vi "MouseWheelEvent.vi"(0 "reference in":refnum<class "LcPictureBox.lvclass">, 5 "error in (no error)":errorcluster) -> (14 "reference out":refnum<class "LcPictureBox.lvclass">, 15 "Event Callback Refnum":refnum<k27>, 16 "MouseWheelEvent":refnum<user-event>, 19 "error out":errorcluster)   [LabVIEW 2020, in "LcPictureBox.lvclass"]
uses:
  LcPictureBox.lvclass
  MouseWheelInfo.ctl
  System.Windows.Forms
  CallBackVIs/CallBack_MouseWheel.vi
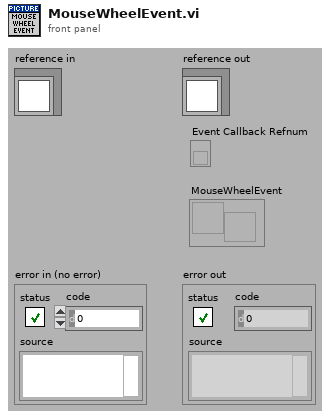
[diagram p1: front panel]
types:
  T1 = typedef "LcPictureBox.lvclass/MouseWheelInfo.ctl" = cluster{"X":i32, "Y":i32, "Button":i32, "Delta":i32, "X(raw)":i32, "Y(raw)":i32}
  T2 = typedef "LcPictureBox.lvclass/ObjectAttributes.ctl" = cluster{"PictureBox":refnum<k24>, "ImageSize":cluster{"Width":i32, "Height":i32}, "PenMemory":map{cluster{"Alpha(100%)":dbl, "Color(Black)":u32, "Pen(Width=1, Solid)":T3}, refnum<k24>}, "GraphicsRef":refnum<k24>, "BrushMemory":map{cluster{"Alpha(100%)":dbl, "Color(Black)":u32}, refnum<k24>}, "Images":refnum<k24>[], "ImageIndex":i32, "BgColor(None)":u32, "LoadedImages":map{string, cluster{"ImageOut":refnum<k24>, "ImageSize":cluster{"Width":i32, "Height":i32}}}, "ColorsMemory":map{cluster{"Alpha(100%)":dbl, "Color(Black)":u32}, refnum<k24>}, "CacheSize":i32, "PictureBoxActiveXReference":refnum<vi>, "Scale":sgl, "Offset":cluster{"x":sgl, "y":sgl}, "zoom_center":cluster{"X":i32, "Y":i32}, "ImagesCreated":refnum<k24>[]}
  T3 = typedef "LcPictureBox.lvclass/Pen.ctl" = cluster{"Width":u16, "Style":enum32{"Solid", "Dash", "Dot", "DashDot", "DashDotDot"}}
  T4 = cluster{"reference out":refnum<class "LcPictureBox.lvclass">, "MouseInfo":refnum<user-event>}
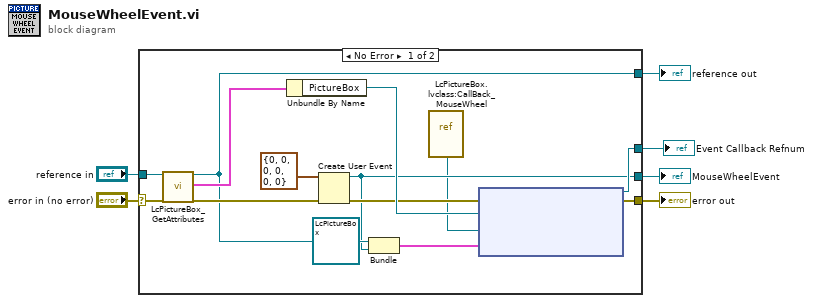
[diagram p0: block diagram]
diagram:
  n1 = case shown="No Error" "error in (no error)" {
    selector: "error in (no error)" -> [w19 w21]
    tunnel: [w13 w21] -> w5
    tunnel: [w10 w20] -> w3
    tunnel: "reference in" -> [w17 w20]
    tunnel: [w9 _] -> w1
    tunnel: [w12 _] -> w2
    frame No Error {
      (unwired) refnum<class "LcPictureBox.lvclass"> refnum ("reference out")
      n2 = call "LcPictureBox_GetAttributes.vi"("reference in"=w17, "error in (no error)"=w19) -> ("reference out"=w10:refnum<class "LcPictureBox.lvclass">, "Data"=w18:T2, "error out"=w14:errorcluster)  [unwired: 14 in, 1 out]
      n3 = Unbundle By Name(w18) -> ("PictureBox"=w16:refnum<k24>)
      n4 = Create User Event(user event datatype=T1 {"X"=0, "Y"=0, "Button"=0, "Delta"=0, "X(raw)"=0, "Y(raw)"=0} ("MouseInfo"), error in=w14) -> (user event=w9:refnum<user-event>, error out=w15:errorcluster)
      n5 = Bundle("reference out"=w10, "MouseInfo"=w9) -> (w7:T4)  [unwired: 1 in]
      n6 = vi-ref "LcPictureBox.lvclass:CallBack_MouseWheel.vi"() -> ("vi reference"=w8:refnum<vi>)
      n7 = node(w15, w16, w8, w7) -> (w12:refnum<k27>, w13:errorcluster)  [unwired: 1 in]
    }
    frame Error {
    }
  }
  "error out" <- w5
  "reference out" <- w3
  "MouseWheelEvent" <- w1
  "Event Callback Refnum" <- w2
